vi "RTC SET Date Time Example.vi"() -> ()   [LabVIEW 2014]
uses:
  QwaveSys_Interface/QwaveSys_Interface.lvlib
  QwaveSys_ESP8266/QwaveSys_ESP8266.lvlib
panel:
  in  "time string":string="19:01:56"
  in  "date string":string="Dec 19 2015"
  # "These two wire for I2C (SDA,SCL) must be connected in order to use onboard RTC with Wemos D1 ESP8266 Board"
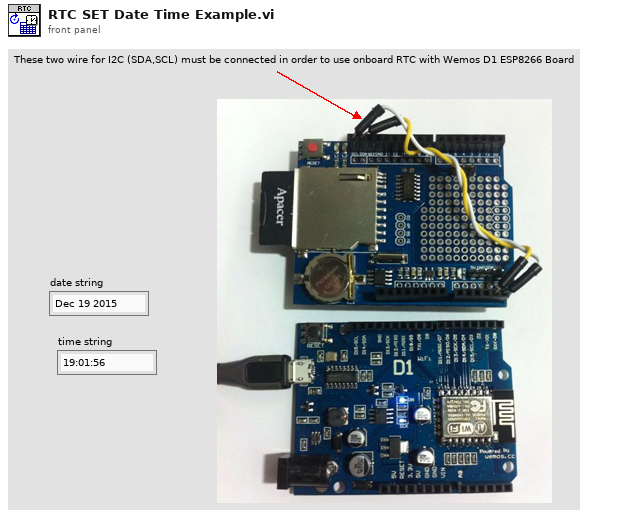
[diagram p1: front panel]
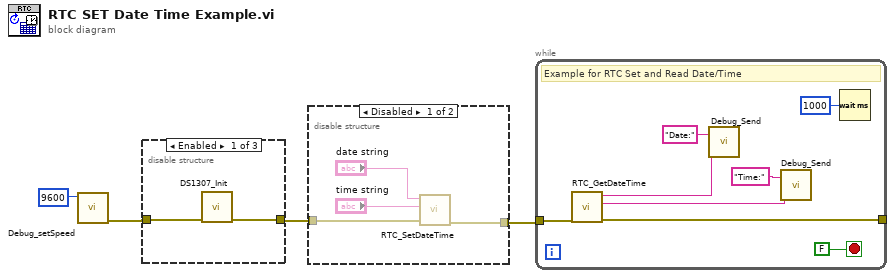
[diagram p0: block diagram]
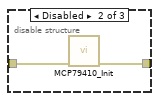
[diagram p3: hidden frame]
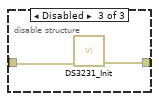
[diagram p4: hidden frame]
diagram:
  n1 = call "Debug_setSpeed.vi"("Speed"=u32 9600) -> ("error out"=w2:errorcluster)  [unwired: 10 in]
  n2 = disable-structure shown="Enabled" {
    disable-tunnel: [w6 w8 w10] -> w1
    disable-tunnel: w2 -> [w5 w7 w9]
    frame Enabled {
      n3 = call "DS1307_Init.vi"("error in (no error)"=w5) -> ("error out"=w6:errorcluster)  [unwired: 10 in]
    }
    frame Disabled {
      n4 = call "MCP79410_Init.vi"("error in (no error)"=w7) -> ("error out"=w8:errorcluster)  [unwired: 10 in]
    }
    frame Disabled {
      n5 = call "DS3231_Init.vi"("error in (no error)"=w9) -> ("error out"=w10:errorcluster)  [unwired: 10 in]
    }
  }
  n6 = disable-structure shown="Disabled" {
    disable-tunnel: [w14 _] -> w3
    disable-tunnel: w1 -> [w13 _]
    frame Disabled {
      n7 = call "RTC_SetDateTime.vi"("error in (no error)"=w13, "time string"="time string", "date string"="date string") -> ("error out"=w14:errorcluster)  [unwired: 8 in]
    }
    frame Enabled {
    }
  }
  n8 = while {
    tunnel: w3 -> [w22]
    tunnel: [w17] -> _
    stop <- FALSE stop-if-true
    # "Example for RTC Set and Read Date/Time"
    n9 = call "RTC_GetDateTime.vi"("error in (no error)"=w22) -> ("error out"=w17:errorcluster, "time string"=w19:string, "date string"=w20:string)  [unwired: 8 in]
    n10 = call "Debug_Send.vi"("Name"="Date:", "DATA"=w20) -> ()  [unwired: 10 in]
    n11 = call "Debug_Send.vi"("Name"="Time:", "DATA"=w19) -> ()  [unwired: 10 in]
    n12 = Wait (ms)(milliseconds to wait=u32 1000) -> ()  [unwired: 1 out]
  }
